vi "Get All Values.vi"(11 "Array 2":refnum<visa-resource-name>[](array[refnum])) -> (2 "Array":dbl[][](array[numeric]), 3 "Array 3":refnum<visa-resource-name>[](array[refnum]))   [LabVIEW 2024]
panel:
  out "read buffer":string
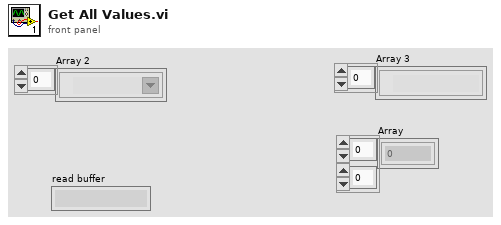
[diagram p1: front panel]
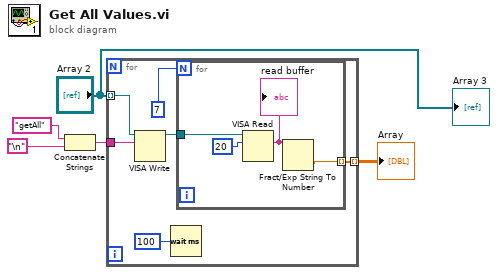
[diagram p0: block diagram]
diagram:
  n1 = Concatenate Strings("getAll" ("string"), "\n") -> (w3:string)
  n2 = for {
    tunnel: [w10] -> w2 mode=indexing
    tunnel: "Array 2" -> [w8] mode=indexing
    tunnel: w3 -> [w7]
    n3 = VISA Write(VISA resource name=w8, write buffer=w7) -> (VISA resource name out=w9:refnum<visa-resource-name>)  [unwired: 1 in, 2 out]
    n4 = Wait (ms)(milliseconds to wait=u32 100) -> ()  [unwired: 1 out]
    n5 = for {
      N: 7 -> [_]
      tunnel: [w12] -> w10 mode=indexing
      tunnel: w9 -> [w14]
      n6 = VISA Read(VISA resource name=w14, byte count=u32 20) -> (read buffer=w13:string)  [unwired: 1 in, 3 out]
      "read buffer" <- w13
      n7 = Fract/Exp String To Number(string=w13) -> (number=w12:dbl)  [unwired: 3 in, 1 out]
    }
  }
  "Array" <- w2
  "Array 3" <- "Array 2"
